vi "Add Bitfile as Dependent File Property.vi"(8 "error in":errorcluster, 10 "Local bitfile path":path, 11 "Device Item Ref":T1=18446744073709551615 format="%.0x") -> (0 "error out":errorcluster, 3 "Device Item Ref out":T1=18446744073709551615 format="%.0x")   [LabVIEW 2019, in "Fuel Injector Analysis Addon System Explorer.lvlib"]
uses:
  Fuel Injector Analysis Addon System Explorer.lvlib
  <vilib>/NI VeriStand/Custom Device API/Custom Device Item Ref.ctl
  <vilib>/NI VeriStand/Custom Device API/Dependent File Optional Info.ctl
  Addon Shared/SubVIs/Constants.vi
  <vilib>/NI VeriStand/Custom Device API/Set Item Property (Dependent File).vi
  <vilib>/NI VeriStand/Custom Device API/Set Item Property (Path).vi
  Addon Shared/Fuel Injector Analysis Addon Shared.lvlib
  <vilib>/NI VeriStand/Custom Device API/Custom Device API.lvlib
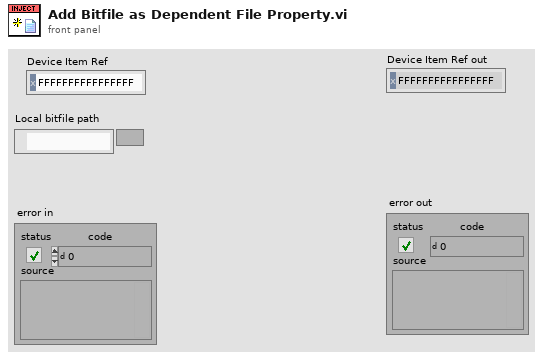
[diagram p1: front panel]
types:
  T1 = typedef "Custom Device API.lvlib/Custom Device Item Ref.ctl" = u64
  T2 = typedef "Custom Device API.lvlib/Dependent File Optional Info.ctl" = cluster{"Version":string, "RTDestination":path, "ForceDownload":bool, "SupportedTarget":string, "MD5":string}
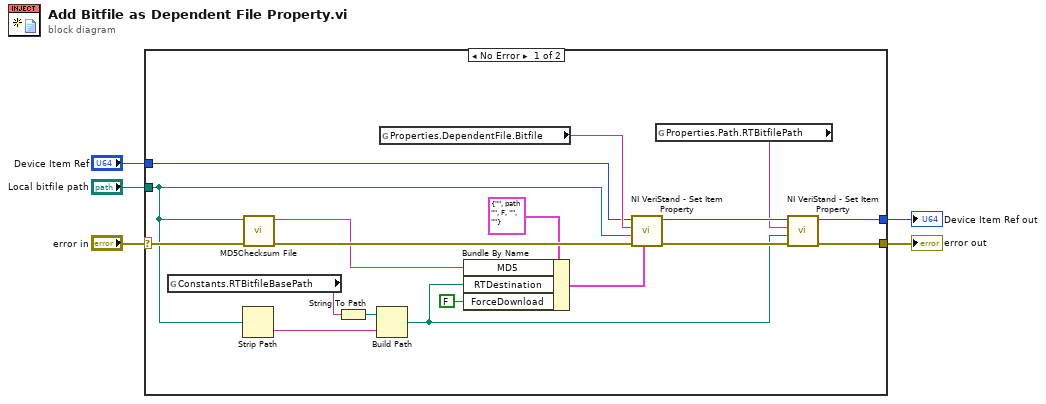
[diagram p0: block diagram]
diagram:
  n1 = case shown="No Error" "error in" {
    selector: "error in" -> [w23 w24]
    tunnel: "Device Item Ref" -> [w13 w25]
    tunnel: "Local bitfile path" -> [w17 _]
    tunnel: [w8 w24] -> w2
    tunnel: [w7 w25] -> w1
    frame No Error {
      n2 = global read "Constants.vi" "Constants.RTBitfileBasePath"() -> (w20:string)
      n3 = Strip Path(path=w17) -> (name=w21:string)  [unwired: 1 out]
      n4 = call <vilib>:"MD5Checksum File.vi"("error in (no error)"=w23, "Path"=w17) -> ("error out"=w22:errorcluster, "MD5 message-digest"=w15:string)  [unwired: 8 in]
      n5 = String To Path(string=w20) -> (path=w19:path)
      n6 = Build Path(base path=w19, name or relative path=w21) -> (appended path=w9:path)
      n7 = global read "Constants.vi" "Properties.DependentFile.Bitfile"() -> (w18:string)
      n8 = Bundle By Name(cluster=T2 {"Version"="", "RTDestination"=path "", "ForceDownload"=FALSE, "SupportedTarget"="", "MD5"=""} ("OptionalInfo"), "MD5"=w15, "RTDestination"=w9, "ForceDownload"=FALSE) -> (w14:T2)
      n9 = call-poly <vilib>:"NI VeriStand - Set Item Property.vi"("OptionalInfo"=w14, "error in (no error)"=w22, "Path"=w17, "Property Name"=w18, "Item Ref in"=w13) -> ("error out"=w11:errorcluster, "Item Ref out"=w12:T1)  [unwired: 4 in, 1 out]
      n10 = global read "Constants.vi" "Properties.Path.RTBitfilePath"() -> (w10:string)
      n11 = call-poly <vilib>:"NI VeriStand - Set Item Property.vi"("error in (no error)"=w11, "Value"=w9, "Property Name"=w10, "Item Ref in"=w12) -> ("error out"=w8:errorcluster, "Item Ref out"=w7:T1)  [unwired: 5 in, 1 out]
    }
    frame Error {
    }
  }
  "error out" <- w2
  "Device Item Ref out" <- w1
